vi "Get Object Names.vi"(11 "tokens in":cluster{"token type":T1, "info":T2}[](array[cluster])) -> (2 "Names":string[](array[string]), 3 "Array":cluster{"match string":string, i32}[](array[cluster]))   [LabVIEW 2019]
uses:
  <vilib>/MultiError/TokenizeJSON/JSON Token Values.ctl
  <vilib>/MultiError/Errors Cluster Multiple Errors/JSON Token Descriptor.ctl
  <vilib>/MultiError/TokenizeJSON/JSON Raw Token Values.ctl
  <vilib>/MultiError/TokenizeJSON/Multi Error Cluster.lvlib
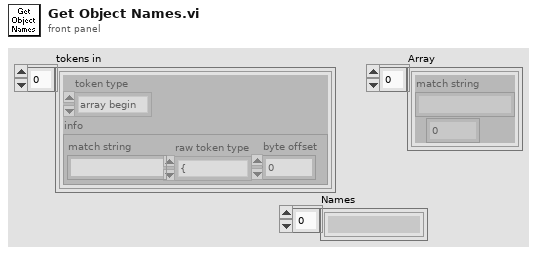
[diagram p1: front panel]
types:
  T1 = typedef "Multi Error Cluster.lvlib/JSON Token Values.ctl" = enum32{"array begin", "array end", "object begin", "object end", "value", "invalid", "name"}
  T2 = typedef "Multi Error Cluster.lvlib/JSON Token Descriptor.ctl" = cluster{"match string":string, "raw token type":T3, "byte offset ":i32}
  T3 = typedef "Multi Error Cluster.lvlib/JSON Raw Token Values.ctl" = enum32{"{", "}", "[", "]", ",", ":", "\"", "number", "string", "true", "false", "null", "invalid"}
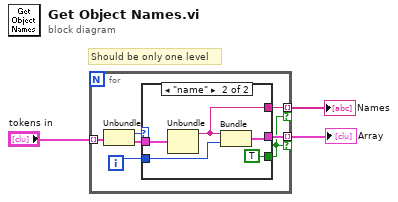
[diagram p0: block diagram]
diagram:
  # "Should be only one level"
  n1 = for {
    tunnel: "tokens in" -> [w10] mode=indexing
    tunnel: [w6] -> w3 mode=indexing if=w4
    tunnel: [w5] -> w1 mode=indexing if=w4
    i -> [w7]
    n2 = Unbundle(w10) -> ("token type"=w9:T1, "info"=w8:T2)
    n3 = case shown="\"name\"" w9 {
      tunnel: w8 -> [_ w15]
      tunnel: w7 -> [_ w14]
      tunnel: [_ w13] -> w6
      tunnel: [_ TRUE] -> w4
      tunnel: [_ w11] -> w5
      frame "array begin", Default {
      }
      frame "name" {
        n4 = Unbundle(w15) -> ("match string"=w11:string)  [unwired: 2 out]
        n5 = Bundle("match string"=w11, w14) -> (w13:cluster{"match string":string, i32})  [unwired: 1 in]
      }
    }
  }
  "Array" <- w3
  "Names" <- w1
